vi "MCSControlPanel.vi"(4 "Register Map\nDefaults":refnum<vi>, 5 "StatusWord0x10Ref":refnum<vi>, 6 "Register Map\nRead Ref":refnum<vi>, 7 "NewRegMapReady":refnum<vi>, 8 "Last Command\nSent Ref":refnum<vi>, 9 "Stop Loop \nRef":refnum<vi>, 10 "error out":errorcluster, 11 "queue out":refnum<queue>) -> ()   [LabVIEW 2012]
panel:
  out "0x10 Status Word Readout":bool[][](array[boolean])
  in  "SYNC In \nVolt Threshold":u16
  out "word33":string
  in  "DIN In Volt \nThreshold":u16
  out "word32":string
  in  "DEMUX In Volt \nThreshold":u16
  out "word31":string
  in  "Power Mon Volt \nRef Threshold":u16
  out "word30":string
  out "wordB":string
  in  "Power Mon In 5 \nDEMUX Select":string(combo)
  in  "Power Mon In 4 \nDEMUX Select":string(combo)
  in  "Power Mon In 3 \nDEMUX Select":string(combo)
  in  "Power Mon In 2 \nDEMUX Select":string(combo)
  in  "Power Mon In 1 \nDEMUX Select":string(combo)
  in  "Power Mon In 0 \nDEMUX Select":string(combo)
  in  "Power Pulse\nReject Config":u16
  in  "Power Mon \nAcc Mode":string(combo)
  in  "Power Mon \nTest Mode":string(combo)
  in  "Power Mon Chan Enable   \n  11    10      9      8       7       6      5       4       3       2      1       0":bool[](array[boolean])
  out "word9":string
  in  "SoftDEMUX \nSelector Enable":bool
  in  "Sync Select 3B":string(combo)
  in  "Sync Select 2B":string(combo)
  in  "Sync Select 1B":string(combo)
  in  "Sync Select 0B":string(combo)
  in  "Sync Select 7":string(combo)
  in  "Sync Select 6":string(combo)
  in  "Sync Select 5":string(combo)
  in  "Sync Select 4":string(combo)
  in  "Sync Select 3A":string(combo)
  in  "Sync Select 2A":string(combo)
  in  "Sync Select 1A":string(combo)
  in  "Sync Select 0A":string(combo)
  in  "Sync Test\nMode Config":u32
  in  "Pulse Period\n(clock cycles -1)":u32
  in  "Channel DEMUX \nSelector":bool
  in  "Channel \nHold Order":bool
  in  "Channel \nTransfer Order":bool
  in  "Throttle Mode":string(combo)
  in  "Sync Test Mode Select":string(combo)
  in  "Data Input Test Mode":string(combo)
  out "Last Command Sent":string
  in  "Send Command, \nmanual entry":string
  in  "Send":bool
  in  "Reset Register Map\nto Defaults":bool
  in  "Sync Enable\n  2       1       0":bool[](array[boolean])
  in  "Channel Enable\n 11     10      9      8       7       6      5        4      3       2       1       0":bool[](array[boolean])
  in  "Reset Profile Accumulator  \n  11     10     9      8       7       6      5       4       3      2       1       0":bool[](array[boolean])
  in  "Counts Per Bin":u16
  in  "User Reset":bool
  in  "Number of Bins":u16
  in  "Profiles Per Histogram":u16
  in  "Time Reset":bool
  in  "Relative Time Step":u32
  in  "Demux Channel Enable\n  3       2       1      0":bool[](array[boolean])
  out "word0":string
  out "word1":string
  out "word2":string
  out "word3":string
  out "word4":string
  out "word5":string
  out "word6":string
  out "word7":string
  out "word8":string
  in  "DIN Polarity \n  7      6        5      4       3       2      1       0":bool[](array[boolean])
  in  "DIN Demux Polarity\n  3       2       1      0":bool[](array[boolean])
  in  "Sync Input Polarity\n  2       1       0":bool[](array[boolean])
  in  "PIN0 Pulse \nDurration Ave 2^N":u16
  out "wordA":string
  in  "PIN1 Pulse \nDurration Ave 2^N":u16
  in  "PIN2 Pulse \nDurration Ave 2^N":u16
  in  "PIN3 Pulse \nDurration Ave 2^N":u16
  in  "PIN4 Pulse \nDurration Ave 2^N":u16
  in  "PIN5 Pulse \nDurration Ave 2^N":u16
  # "word00"
  # "word30"
  # "valid range (0-65535)"
  # "word01"
  # "word02"
  # "word03"
  # "word04"
  # "word31"
  # "valid range (2-4095)"
  # "valid range (2-4095)"
  # "valid range (1-32,767)"
  # "valid range (0-65535)"
  # "word32"
  # "word05"
  # "valid range (0-65535)"
  # "7\n15\n23\n31"
  # "0\n8\n16\n24"
  # "word33"
  # "word06"
  # "valid range (0-65535)"
  # "valid range (0-255)"
  # "valid range (0-63)"
  # "word07"
  # "word08"
  # "word09"
  # "valid range (0-33,554,431)"
  # "valid range (0-256)"
  # "word0A"
  # "word0B"
  # "Expert Use Only"
  # "N=valid range (0-15)"
  # "N=valid range (0-15)"
  # "N=valid range (0-15)"
  # "N=valid range (0-15)"
  # "N=valid range (0-15)"
  # "N=valid range (0-15)"
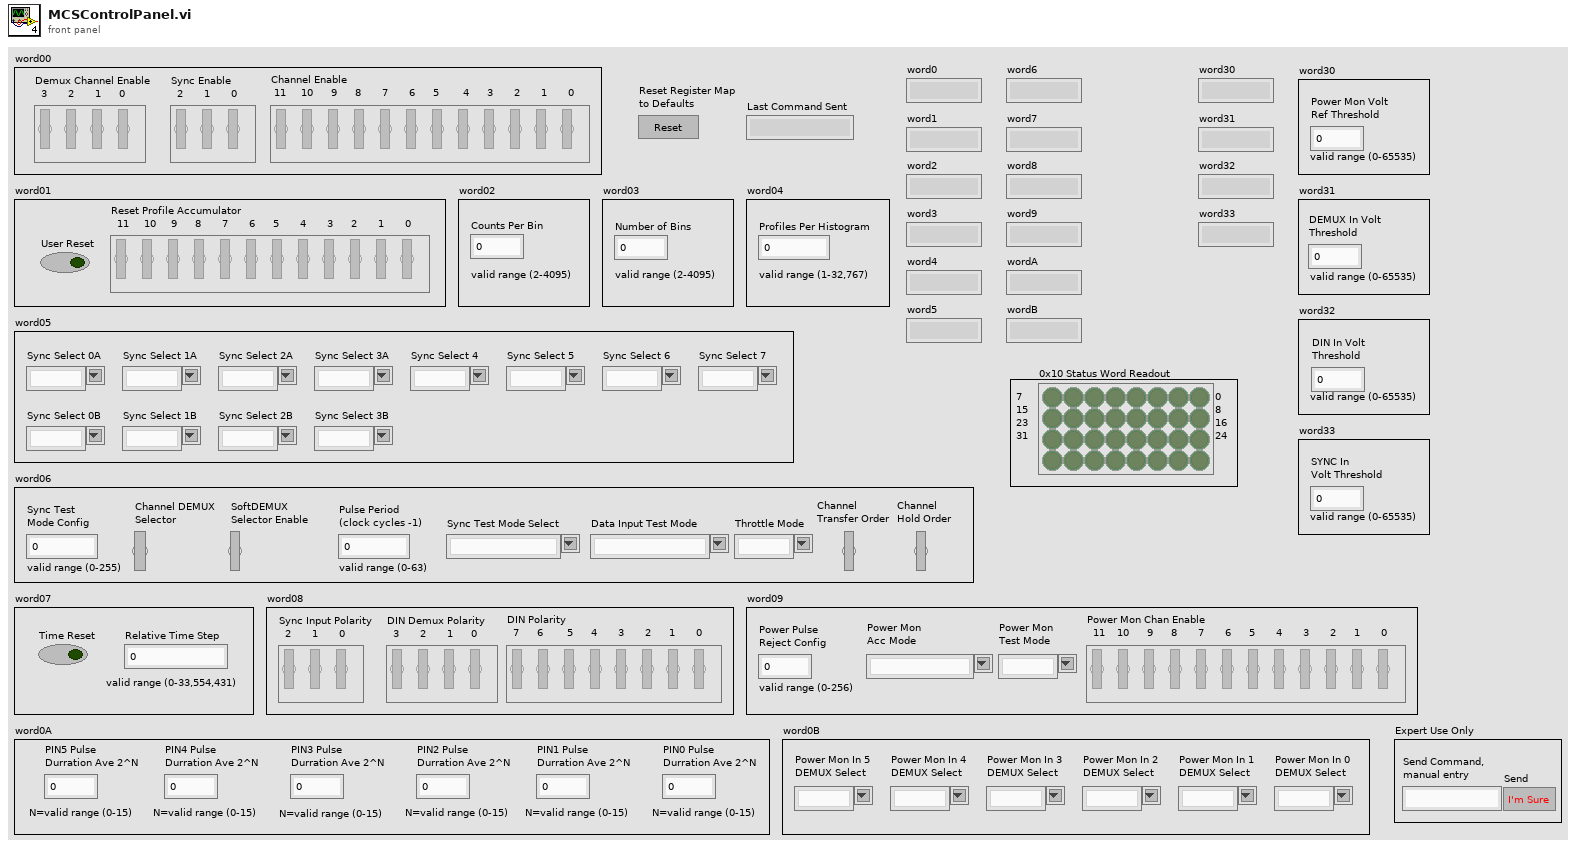
[diagram p1: front panel]
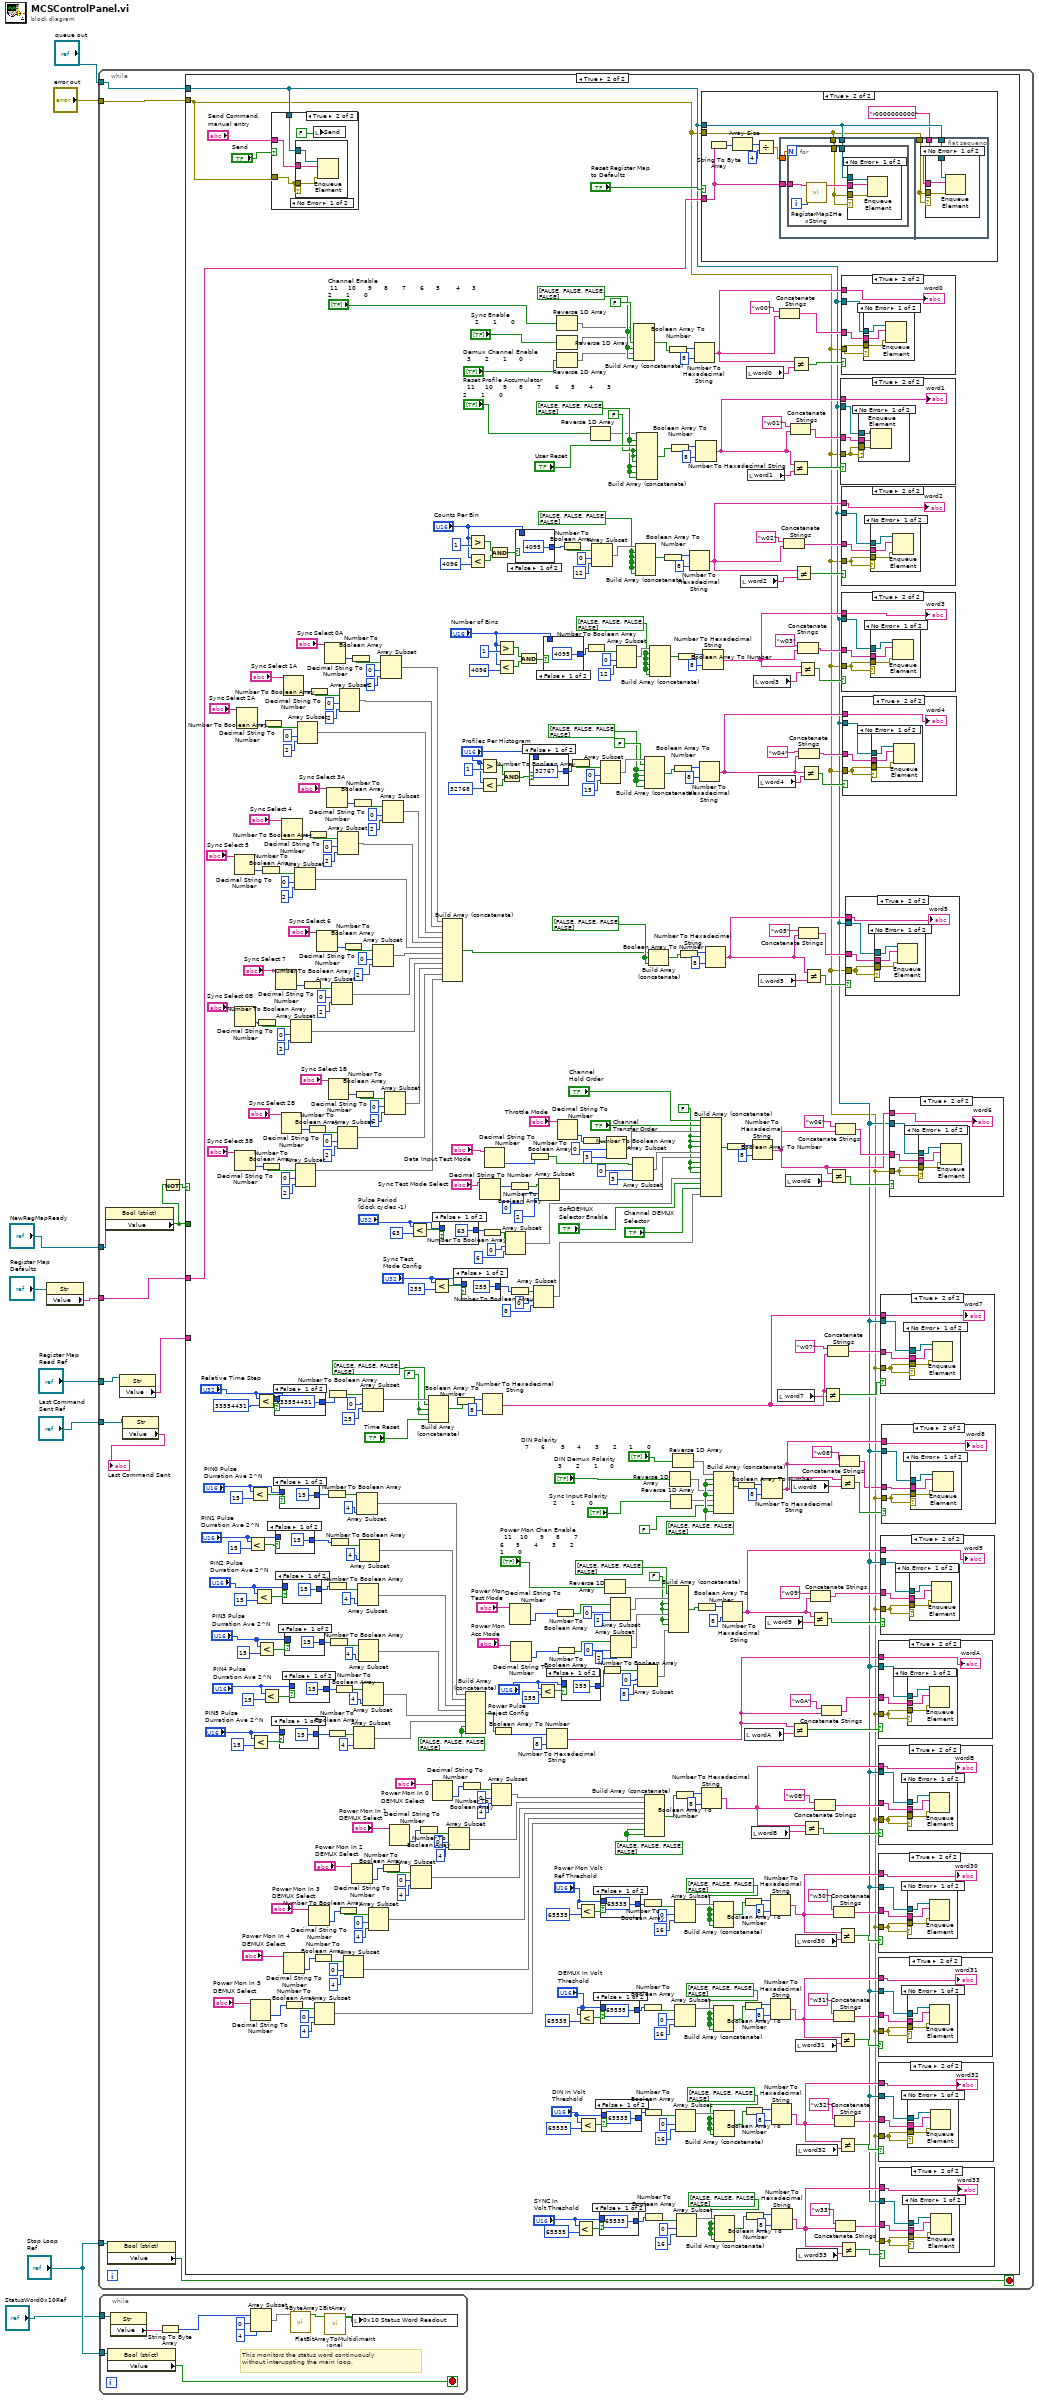
[diagram p0: block diagram]
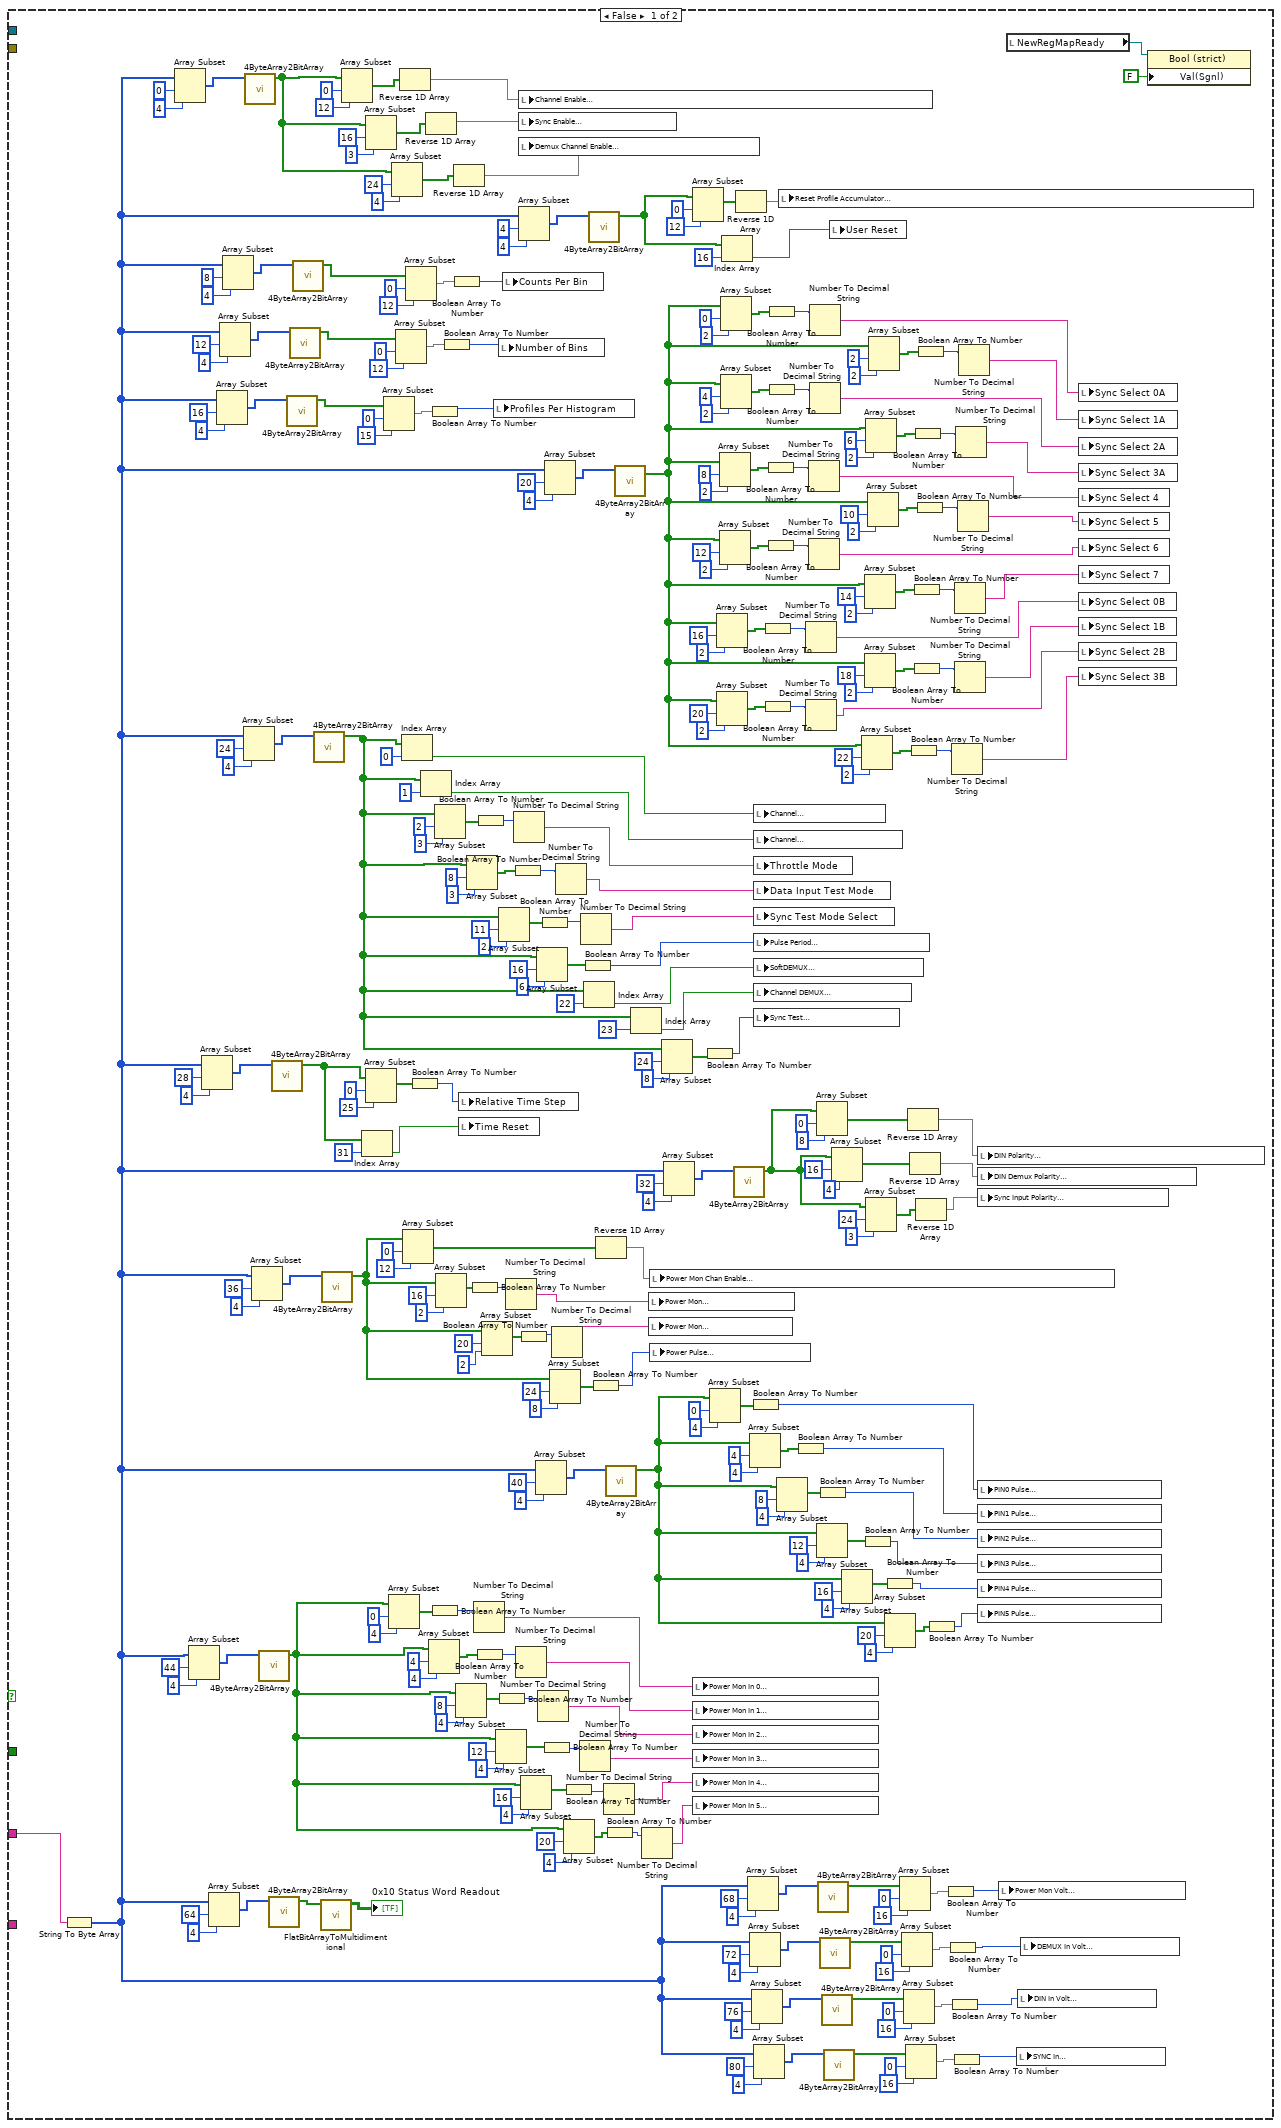
[diagram p2: hidden frame]
diagram:
  n1 = property class="Str"(reference="Register Map\nDefaults") -> ("Value"=w3:string)  [unwired: 1 in, 2 out]
  n2 = while {
    tunnel: "queue out" -> [w21]
    tunnel: "error out" -> [w20]
    tunnel: "Stop Loop \nRef" -> [w19]
    tunnel: "Last Command\nSent Ref" -> [w15]
    tunnel: "Register Map\nRead Ref" -> [w16]
    tunnel: w3 -> [w12]
    tunnel: "NewRegMapReady" -> [w13]
    stop <- w18 stop-if-true
    n3 = property class="Bool (strict)"(reference=w13) -> ("Value"=w10:bool)  [unwired: 1 in, 2 out]
    n4 = property class="Bool (strict)"(reference=w19) -> ("Value"=w18:bool)  [unwired: 1 in, 2 out]
    n5 = property class="Str"(reference=w16) -> ("Value"=w14:string)  [unwired: 1 in, 2 out]
    n6 = property class="Str"(reference=w15) -> ("Value"=→"Last Command Sent":string)  [unwired: 1 in, 2 out]
    n7 = Not(x=w10) -> (.not. x?=w11:bool)
    n8 = case shown="True" w11 {
      tunnel: w21 -> [_ w409]
      tunnel: w20 -> [_ w337]
      tunnel: w14 -> [_ _]
      tunnel: w12 -> [w44 w578]
      tunnel: w10 -> [_ _]
      frame False {
        n9 = String To Byte Array(string=w44) -> (unsigned byte array=w41:u8[])
        n10 = Array Subset(array=w41, index=0, length=4) -> (w290:u8[])
        n11 = Array Subset(array=w41, index=44, length=4) -> (w108:u8[])
        n12 = Array Subset(array=w41, index=28, length=4) -> (w296:u8[])
        n13 = Array Subset(array=w41, index=64, length=4) -> (w40:u8[])
        n14 = Array Subset(array=w41, index=16, length=4) -> (w305:u8[])
        n15 = Array Subset(array=w41, index=12, length=4) -> (w308:u8[])
        n16 = Array Subset(array=w41, index=8, length=4) -> (w311:u8[])
        n17 = Array Subset(array=w41, index=24, length=4) -> (w299:u8[])
        n18 = call "4ByteArray2BitArray.vi"("array"=w290) -> ("Array"=w136:bool[])  [unwired: 10 in]
        n19 = Array Subset(array=w41, index=36, length=4) -> (w130:u8[])
        n20 = call "4ByteArray2BitArray.vi"("array"=w108) -> ("Array"=w89:bool[])  [unwired: 10 in]
        n21 = call "4ByteArray2BitArray.vi"("array"=w40) -> ("Array"=w25:bool[])  [unwired: 10 in]
        n22 = call "4ByteArray2BitArray.vi"("array"=w296) -> ("Array"=w255:bool[])  [unwired: 10 in]
        n23 = call "4ByteArray2BitArray.vi"("array"=w305) -> ("Array"=w157:bool[])  [unwired: 10 in]
        n24 = call "4ByteArray2BitArray.vi"("array"=w308) -> ("Array"=w152:bool[])  [unwired: 10 in]
        n25 = call "4ByteArray2BitArray.vi"("array"=w311) -> ("Array"=w147:bool[])  [unwired: 10 in]
        n26 = call "4ByteArray2BitArray.vi"("array"=w299) -> ("Array"=w135:bool[])  [unwired: 10 in]
        n27 = call "FlatBitArrayToMultidimentional.vi"("Array in"=w25) -> ("Array out"=→"0x10 Status Word Readout":bool[][])  [unwired: 10 in]
        n28 = call "4ByteArray2BitArray.vi"("array"=w130) -> ("Array"=w117:bool[])  [unwired: 10 in]
        n29 = Array Subset(array=w136, index=0, length=12) -> (w38:bool[])
        n30 = Index Array(array=w255, index=31) -> (element=w253:bool)
        n31 = Array Subset(array=w136, index=16, length=3) -> (w36:bool[])
        n32 = Array Subset(array=w255, index=0, length=25) -> (w251:bool[])
        n33 = Array Subset(array=w157, index=0, length=15) -> (w158:bool[])
        n34 = Array Subset(array=w89, index=0, length=4) -> (w94:bool[])
        n35 = Array Subset(array=w136, index=24, length=4) -> (w34:bool[])
        n36 = Array Subset(array=w152, index=0, length=12) -> (w153:bool[])
        n37 = Reverse 1D Array(array=w38) -> (reversed array=w39:bool[])
        n38 = Index Array(array=w135, index=0) -> (element=w233:bool)
        n39 = Array Subset(array=w117, index=0, length=12) -> (w26:bool[])
        n40 = Array Subset(array=w147, index=0, length=12) -> (w148:bool[])
        n41 = Boolean Array To Number(Boolean array=w251) -> (number=w252:u32)
        n42 = Index Array(array=w135, index=1) -> (element=w232:bool)
        n43 = Reverse 1D Array(array=w36) -> (reversed array=w37:bool[])
        n44 = Array Subset(array=w89, index=4, length=4) -> (w95:bool[])
        n45 = Boolean Array To Number(Boolean array=w158) -> (number=w156:u32)
        n46 = Boolean Array To Number(Boolean array=w94) -> (number=w88:u32)
        n47 = Array Subset(array=w135, index=2, length=3) -> (w239:bool[])
        n48 = Array Subset(array=w117, index=16, length=2) -> (w126:bool[])
        n49 = Boolean Array To Number(Boolean array=w153) -> (number=w151:u32)
        n50 = Boolean Array To Number(Boolean array=w148) -> (number=w146:u32)
        n51 = Reverse 1D Array(array=w34) -> (reversed array=w35:bool[])
        n52 = Array Subset(array=w89, index=8, length=4) -> (w93:bool[])
        n53 = local write "Relative Time Step"(w252) -> ()
        n54 = local write "Time Reset"(w253) -> ()
        n55 = Array Subset(array=w135, index=8, length=3) -> (w240:bool[])
        n56 = Boolean Array To Number(Boolean array=w126) -> (number=w125:u32)
        n57 = Number To Decimal String(number=w88) -> (decimal integer string=w77:string)  [unwired: 1 in]
        n58 = Boolean Array To Number(Boolean array=w95) -> (number=w87:u32)
        n59 = Boolean Array To Number(Boolean array=w239) -> (number=w231:u32)
        n60 = Array Subset(array=w117, index=20, length=2) -> (w122:bool[])
        n61 = local write "Profiles Per Histogram"(w156) -> ()
        n62 = Array Subset(array=w89, index=12, length=4) -> (w92:bool[])
        n63 = Boolean Array To Number(Boolean array=w93) -> (number=w86:u32)
        n64 = local write "Number of Bins"(w151) -> ()
        n65 = Array Subset(array=w135, index=11, length=2) -> (w238:bool[])
        n66 = local write "Counts Per Bin"(w146) -> ()
        n67 = Number To Decimal String(number=w125) -> (decimal integer string=w124:string)  [unwired: 1 in]
        n68 = Boolean Array To Number(Boolean array=w240) -> (number=w229:u32)
        n69 = Number To Decimal String(number=w231) -> (decimal integer string=w230:string)  [unwired: 1 in]
        n70 = Number To Decimal String(number=w87) -> (decimal integer string=w78:string)  [unwired: 1 in]
        n71 = local write "Channel Enable\n 11     10      9      8       7       6      5        4      3       2       1       0"(w39) -> ()
        n72 = local write "Sync Enable\n  2       1       0"(w37) -> ()
        n73 = local write "Demux Channel Enable\n  3       2       1      0"(w35) -> ()
        n74 = Array Subset(array=w41, index=4, length=4) -> (w314:u8[])
        n75 = Boolean Array To Number(Boolean array=w122) -> (number=w121:u32)
        n76 = Array Subset(array=w89, index=16, length=4) -> (w91:bool[])
        n77 = Array Subset(array=w41, index=40, length=4) -> (w317:u8[])
        n78 = Array Subset(array=w135, index=16, length=6) -> (w237:bool[])
        n79 = Number To Decimal String(number=w86) -> (decimal integer string=w79:string)  [unwired: 1 in]
        n80 = Boolean Array To Number(Boolean array=w238) -> (number=w227:u32)
        n81 = Boolean Array To Number(Boolean array=w92) -> (number=w84:u32)
        n82 = Array Subset(array=w41, index=20, length=4) -> (w302:u8[])
        n83 = Array Subset(array=w117, index=24, length=8) -> (w118:bool[])
        n84 = Number To Decimal String(number=w121) -> (decimal integer string=w120:string)  [unwired: 1 in]
        n85 = Number To Decimal String(number=w229) -> (decimal integer string=w228:string)  [unwired: 1 in]
        n86 = Boolean Array To Number(Boolean array=w91) -> (number=w85:u32)
        n87 = Array Subset(array=w89, index=20, length=4) -> (w90:bool[])
        n88 = Number To Decimal String(number=w84) -> (decimal integer string=w80:string)  [unwired: 1 in]
        n89 = Number To Decimal String(number=w227) -> (decimal integer string=w226:string)  [unwired: 1 in]
        n90 = Boolean Array To Number(Boolean array=w237) -> (number=w223:u32)
        n91 = Index Array(array=w135, index=22) -> (element=w133:bool)
        n92 = call "4ByteArray2BitArray.vi"("array"=w314) -> ("Array"=w142:bool[])  [unwired: 10 in]
        n93 = Boolean Array To Number(Boolean array=w118) -> (number=w116:u32)
        n94 = Reverse 1D Array(array=w26) -> (reversed array=w27:bool[])
        n95 = Number To Decimal String(number=w85) -> (decimal integer string=w81:string)  [unwired: 1 in]
        n96 = Boolean Array To Number(Boolean array=w90) -> (number=w83:u32)
        n97 = call "4ByteArray2BitArray.vi"("array"=w317) -> ("Array"=w277:bool[])  [unwired: 10 in]
        n98 = call "4ByteArray2BitArray.vi"("array"=w302) -> ("Array"=w173:bool[])  [unwired: 10 in]
        n99 = Index Array(array=w135, index=23) -> (element=w224:bool)
        n100 = Number To Decimal String(number=w83) -> (decimal integer string=w82:string)  [unwired: 1 in]
        n101 = local write "Power Mon \nTest Mode"(w124) -> ()
        n102 = local write "Power Mon \nAcc Mode"(w120) -> ()
        n103 = local write "Power Mon Chan Enable   \n  11    10      9      8       7       6      5       4       3       2      1       0"(w27) -> ()
        n104 = local write "Power Pulse\nReject Config"(w116) -> ()
        n105 = Array Subset(array=w135, index=24, length=8) -> (w236:bool[])
        n106 = Array Subset(array=w41, index=32, length=4) -> (w293:u8[])
        n107 = Array Subset(array=w142, index=0, length=12) -> (w32:bool[])
        n108 = local write "Power Mon In 0 \nDEMUX Select"(w77) -> ()
        n109 = local write "Power Mon In 1 \nDEMUX Select"(w78) -> ()
        n110 = local write "Power Mon In 2 \nDEMUX Select"(w79) -> ()
        n111 = local write "Power Mon In 3 \nDEMUX Select"(w80) -> ()
        n112 = local write "Power Mon In 4 \nDEMUX Select"(w81) -> ()
        n113 = local write "Power Mon In 5 \nDEMUX Select"(w82) -> ()
        n114 = Boolean Array To Number(Boolean array=w236) -> (number=w222:u32)
        n115 = Array Subset(array=w277, index=0, length=4) -> (w274:bool[])
        n116 = Array Subset(array=w173, index=16, length=2) -> (w187:bool[])
        n117 = Array Subset(array=w173, index=20, length=2) -> (w179:bool[])
        n118 = Array Subset(array=w173, index=8, length=2) -> (w203:bool[])
        n119 = Array Subset(array=w173, index=12, length=2) -> (w195:bool[])
        n120 = Array Subset(array=w173, index=0, length=2) -> (w219:bool[])
        n121 = Array Subset(array=w173, index=4, length=2) -> (w211:bool[])
        n122 = Index Array(array=w142, index=16) -> (element=w141:bool)
        n123 = call "4ByteArray2BitArray.vi"("array"=w293) -> ("Array"=w258:bool[])  [unwired: 10 in]
        n124 = Reverse 1D Array(array=w32) -> (reversed array=w33:bool[])
        n125 = Array Subset(array=w41, index=68, length=4) -> (w74:u8[])
        n126 = Array Subset(array=w277, index=4, length=4) -> (w276:bool[])
        n127 = Array Subset(array=w41, index=72, length=4) -> (w67:u8[])
        n128 = Boolean Array To Number(Boolean array=w274) -> (number=w273:u32)
        n129 = Array Subset(array=w41, index=76, length=4) -> (w60:u8[])
        n130 = local write "Channel \nHold Order"(w233) -> ()
        n131 = local write "Channel \nTransfer Order"(w232) -> ()
        n132 = local write "Throttle Mode"(w230) -> ()
        n133 = local write "Data Input Test Mode"(w228) -> ()
        n134 = local write "Sync Test Mode Select"(w226) -> ()
        n135 = local write "Pulse Period\n(clock cycles -1)"(w223) -> ()
        n136 = local write "SoftDEMUX \nSelector Enable"(w133) -> ()
        n137 = local write "Channel DEMUX \nSelector"(w224) -> ()
        n138 = local write "Sync Test\nMode Config"(w222) -> ()
        n139 = Array Subset(array=w41, index=80, length=4) -> (w53:u8[])
        n140 = Boolean Array To Number(Boolean array=w187) -> (number=w186:u32)
        n141 = Boolean Array To Number(Boolean array=w179) -> (number=w178:u32)
        n142 = Boolean Array To Number(Boolean array=w203) -> (number=w202:u32)
        n143 = Boolean Array To Number(Boolean array=w195) -> (number=w194:u32)
        n144 = Boolean Array To Number(Boolean array=w219) -> (number=w218:u32)
        n145 = Boolean Array To Number(Boolean array=w211) -> (number=w210:u32)
        n146 = Array Subset(array=w277, index=8, length=4) -> (w271:bool[])
        n147 = local write "Reset Profile Accumulator  \n  11     10     9      8       7       6      5       4       3      2       1       0"(w33) -> ()
        n148 = Boolean Array To Number(Boolean array=w276) -> (number=w275:u32)
        n149 = Number To Decimal String(number=w186) -> (decimal integer string=w164:string)  [unwired: 1 in]
        n150 = Number To Decimal String(number=w178) -> (decimal integer string=w162:string)  [unwired: 1 in]
        n151 = Number To Decimal String(number=w202) -> (decimal integer string=w168:string)  [unwired: 1 in]
        n152 = Number To Decimal String(number=w194) -> (decimal integer string=w166:string)  [unwired: 1 in]
        n153 = Number To Decimal String(number=w218) -> (decimal integer string=w172:string)  [unwired: 1 in]
        n154 = Number To Decimal String(number=w210) -> (decimal integer string=w170:string)  [unwired: 1 in]
        n155 = Array Subset(array=w258, index=0, length=8) -> (w28:bool[])
        n156 = Array Subset(array=w277, index=12, length=4) -> (w270:bool[])
        n157 = Boolean Array To Number(Boolean array=w271) -> (number=w272:u32)
        n158 = call "4ByteArray2BitArray.vi"("array"=w74) -> ("Array"=w70:bool[])  [unwired: 10 in]
        n159 = call "4ByteArray2BitArray.vi"("array"=w67) -> ("Array"=w63:bool[])  [unwired: 10 in]
        n160 = call "4ByteArray2BitArray.vi"("array"=w60) -> ("Array"=w56:bool[])  [unwired: 10 in]
        n161 = call "4ByteArray2BitArray.vi"("array"=w53) -> ("Array"=w49:bool[])  [unwired: 10 in]
        n162 = local write "User Reset"(w141) -> ()
        n163 = Array Subset(array=w258, index=16, length=4) -> (w29:bool[])
        n164 = Array Subset(array=w277, index=16, length=4) -> (w269:bool[])
        n165 = Array Subset(array=w173, index=22, length=2) -> (w175:bool[])
        n166 = Boolean Array To Number(Boolean array=w270) -> (number=w265:u32)
        n167 = Array Subset(array=w173, index=14, length=2) -> (w191:bool[])
        n168 = Array Subset(array=w173, index=18, length=2) -> (w183:bool[])
        n169 = Array Subset(array=w173, index=6, length=2) -> (w207:bool[])
        n170 = Array Subset(array=w258, index=24, length=3) -> (w30:bool[])
        n171 = Array Subset(array=w173, index=10, length=2) -> (w199:bool[])
        n172 = Array Subset(array=w173, index=2, length=2) -> (w215:bool[])
        n173 = Boolean Array To Number(Boolean array=w269) -> (number=w266:u32)
        n174 = Array Subset(array=w277, index=20, length=4) -> (w268:bool[])
        n175 = Array Subset(array=w70, index=0, length=16) -> (w71:bool[])
        n176 = Array Subset(array=w63, index=0, length=16) -> (w64:bool[])
        n177 = Array Subset(array=w56, index=0, length=16) -> (w57:bool[])
        n178 = Array Subset(array=w49, index=0, length=16) -> (w50:bool[])
        n179 = Reverse 1D Array(array=w28) -> (reversed array=w31:bool[])
        n180 = Boolean Array To Number(Boolean array=w175) -> (number=w174:u32)
        n181 = Reverse 1D Array(array=w29) -> (reversed array=w23:bool[])
        n182 = Boolean Array To Number(Boolean array=w191) -> (number=w190:u32)
        n183 = Boolean Array To Number(Boolean array=w183) -> (number=w182:u32)
        n184 = Boolean Array To Number(Boolean array=w207) -> (number=w206:u32)
        n185 = Boolean Array To Number(Boolean array=w199) -> (number=w198:u32)
        n186 = Boolean Array To Number(Boolean array=w215) -> (number=w214:u32)
        n187 = Reverse 1D Array(array=w30) -> (reversed array=w22:bool[])
        n188 = Boolean Array To Number(Boolean array=w268) -> (number=w267:u32)
        n189 = Boolean Array To Number(Boolean array=w71) -> (number=w48:u32)
        n190 = Boolean Array To Number(Boolean array=w64) -> (number=w47:u32)
        n191 = Boolean Array To Number(Boolean array=w57) -> (number=w46:u32)
        n192 = Number To Decimal String(number=w174) -> (decimal integer string=w161:string)  [unwired: 1 in]
        n193 = Boolean Array To Number(Boolean array=w50) -> (number=w45:u32)
        n194 = Number To Decimal String(number=w190) -> (decimal integer string=w165:string)  [unwired: 1 in]
        n195 = Number To Decimal String(number=w182) -> (decimal integer string=w163:string)  [unwired: 1 in]
        n196 = Number To Decimal String(number=w206) -> (decimal integer string=w169:string)  [unwired: 1 in]
        n197 = Number To Decimal String(number=w198) -> (decimal integer string=w167:string)  [unwired: 1 in]
        n198 = Number To Decimal String(number=w214) -> (decimal integer string=w171:string)  [unwired: 1 in]
        n199 = local write "DIN Polarity \n  7      6        5      4       3       2      1       0"(w31) -> ()
        n200 = local write "DIN Demux Polarity\n  3       2       1      0"(w23) -> ()
        n201 = local write "Sync Input Polarity\n  2       1       0"(w22) -> ()
        n202 = local write "PIN0 Pulse \nDurration Ave 2^N"(w273) -> ()
        n203 = local write "PIN1 Pulse \nDurration Ave 2^N"(w275) -> ()
        n204 = local write "PIN2 Pulse \nDurration Ave 2^N"(w272) -> ()
        n205 = local write "PIN3 Pulse \nDurration Ave 2^N"(w265) -> ()
        n206 = local write "PIN4 Pulse \nDurration Ave 2^N"(w266) -> ()
        n207 = local write "PIN5 Pulse \nDurration Ave 2^N"(w267) -> ()
        n208 = local write "Power Mon Volt \nRef Threshold"(w48) -> ()
        n209 = local read "NewRegMapReady"() -> (w112:refnum<vi>)
        n210 = local write "SYNC In \nVolt Threshold"(w45) -> ()
        n211 = local write "DIN In Volt \nThreshold"(w46) -> ()
        n212 = local write "DEMUX In Volt \nThreshold"(w47) -> ()
        n213 = local write "Sync Select 0A"(w172) -> ()
        n214 = local write "Sync Select 1A"(w171) -> ()
        n215 = local write "Sync Select 2A"(w170) -> ()
        n216 = local write "Sync Select 3A"(w169) -> ()
        n217 = local write "Sync Select 4"(w168) -> ()
        n218 = local write "Sync Select 5"(w167) -> ()
        n219 = local write "Sync Select 6"(w166) -> ()
        n220 = local write "Sync Select 7"(w165) -> ()
        n221 = local write "Sync Select 0B"(w164) -> ()
        n222 = local write "Sync Select 1B"(w163) -> ()
        n223 = local write "Sync Select 2B"(w162) -> ()
        n224 = local write "Sync Select 3B"(w161) -> ()
        n225 = property class="Bool (strict)"(reference=w112, "Val(Sgnl)"=FALSE ("Value (Signaling)")) -> ()  [unwired: 1 in, 2 out]
      }
      frame True {
        w410 = bool[] [FALSE, FALSE, FALSE, FALSE] ("appended array")
        w423 = bool[] [FALSE, FALSE, FALSE, FALSE] ("appended array")
        w436 = bool[] [FALSE, FALSE, FALSE, FALSE] ("appended array")
        w449 = bool[] [FALSE, FALSE, FALSE, FALSE] ("appended array")
        w508 = bool[] [FALSE, FALSE, FALSE, FALSE] ("appended array")
        w407 = FALSE ("Read Register")
        w726 = bool[] [FALSE, FALSE, FALSE, FALSE] ("appended array")
        w744 = bool[] [FALSE, FALSE, FALSE, FALSE] ("appended array")
        w746 = FALSE ("Read Register")
        w687 = FALSE ("Read Register")
        w751 = bool[] [FALSE, FALSE, FALSE, FALSE] ("appended array")
        w610 = bool[] [FALSE, FALSE, FALSE, FALSE] ("appended array")
        w749 = bool[] [FALSE, FALSE, FALSE, FALSE] ("appended array")
        w750 = bool[] [FALSE, FALSE, FALSE, FALSE] ("appended array")
        w762 = FALSE ("Read Register")
        w761 = bool[] [FALSE, FALSE, FALSE, FALSE] ("appended array")
        w764 = bool[] [FALSE, FALSE, FALSE, FALSE] ("appended array")
        n226 = Decimal String To Number(string="Sync Select 5") -> (number=w654:i32)  [unwired: 2 in, 1 out]
        n227 = Decimal String To Number(string="Sync Select 0B") -> (number=w639:i32)  [unwired: 2 in, 1 out]
        n228 = Decimal String To Number(string="Sync Select 3B") -> (number=w624:i32)  [unwired: 2 in, 1 out]
        n229 = Decimal String To Number(string="Sync Select 2A") -> (number=w669:i32)  [unwired: 2 in, 1 out]
        n230 = Less?(x="PIN1 Pulse \nDurration Ave 2^N", y=u16 15) -> (x < y?=w371:bool)
        n231 = Less?(x="PIN0 Pulse \nDurration Ave 2^N", y=u16 15) -> (x < y?=w377:bool)
        n232 = Decimal String To Number(string="Power Mon In 5 \nDEMUX Select") -> (number=w511:i32)  [unwired: 2 in, 1 out]
        n233 = Less?(x="PIN5 Pulse \nDurration Ave 2^N", y=u16 15) -> (x < y?=w382:bool)
        n234 = Less?(x="PIN2 Pulse \nDurration Ave 2^N", y=u16 15) -> (x < y?=w375:bool)
        n235 = Less?(x="Relative Time Step", y=u64 33554431) -> (x < y?=w339:bool)
        n236 = Number To Boolean Array(number=w639) -> (Boolean array=w641:bool[])
        n237 = Less?(x="PIN3 Pulse \nDurration Ave 2^N", y=u16 15) -> (x < y?=w373:bool)
        n238 = Number To Boolean Array(number=w654) -> (Boolean array=w656:bool[])
        n239 = Number To Boolean Array(number=w624) -> (Boolean array=w626:bool[])
        n240 = Less?(x="PIN4 Pulse \nDurration Ave 2^N", y=u16 15) -> (x < y?=w379:bool)
        n241 = Number To Boolean Array(number=w669) -> (Boolean array=w671:bool[])
        n242 = case shown="True" "Send" {
          tunnel: "Send Command, \nmanual entry" -> [_ w953]
          tunnel: w409 -> [_ w952]
          tunnel: w337 -> [_ w950]
          frame False {
          }
          frame True {
            n243 = case shown="No Error" w950 {
              tunnel: w953 -> [w956 _]
              tunnel: w950 -> [w955 _]
              tunnel: w952 -> [w954 _]
              frame No Error {
                n244 = Enqueue Element(queue=w954, element=w956, error in (no error)=w955) -> ()  [unwired: 1 in, 3 out]
              }
              frame Error {
              }
            }
            n245 = local write "Send"(FALSE ("Send")) -> ()
          }
        }
        n246 = case shown="False" w339 {
          tunnel: [u64 33554431 ("Counts Per Bin") w783] -> w328
          tunnel: "Relative Time Step" -> [_ w783]
          frame False {
          }
          frame True {
          }
        }
        n247 = case shown="False" w371 {
          tunnel: [u16 15 ("Counts Per Bin") w795] -> w364
          tunnel: "PIN1 Pulse \nDurration Ave 2^N" -> [_ w795]
          frame False {
          }
          frame True {
          }
        }
        n248 = Decimal String To Number(string="Sync Select 7") -> (number=w644:i32)  [unwired: 2 in, 1 out]
        n249 = case shown="False" w382 {
          tunnel: [u16 15 ("Counts Per Bin") w805] -> w383
          tunnel: "PIN5 Pulse \nDurration Ave 2^N" -> [_ w805]
          frame False {
          }
          frame True {
          }
        }
        n250 = case shown="False" w377 {
          tunnel: [u16 15 ("Counts Per Bin") w801] -> w361
          tunnel: "PIN0 Pulse \nDurration Ave 2^N" -> [_ w801]
          frame False {
          }
          frame True {
          }
        }
        n251 = Decimal String To Number(string="Sync Select 2B") -> (number=w629:i32)  [unwired: 2 in, 1 out]
        n252 = Decimal String To Number(string="Sync Select 4") -> (number=w659:i32)  [unwired: 2 in, 1 out]
        n253 = case shown="False" w375 {
          tunnel: [u16 15 ("Counts Per Bin") w799] -> w366
          tunnel: "PIN2 Pulse \nDurration Ave 2^N" -> [_ w799]
          frame False {
          }
          frame True {
          }
        }
        n254 = Decimal String To Number(string="Sync Select 1A") -> (number=w674:i32)  [unwired: 2 in, 1 out]
        n255 = Decimal String To Number(string="Power Mon In 4 \nDEMUX Select") -> (number=w521:i32)  [unwired: 2 in, 1 out]
        n256 = Number To Boolean Array(number=w511) -> (Boolean array=w512:bool[])
        n257 = case shown="False" w373 {
          tunnel: [u16 15 ("Counts Per Bin") w797] -> w368
          tunnel: "PIN3 Pulse \nDurration Ave 2^N" -> [_ w797]
          frame False {
          }
          frame True {
          }
        }
        n258 = case shown="False" w379 {
          tunnel: [u16 15 ("Counts Per Bin") w803] -> w369
          tunnel: "PIN4 Pulse \nDurration Ave 2^N" -> [_ w803]
          frame False {
          }
          frame True {
          }
        }
        n259 = Array Subset(array=w641, index=0, length=2) -> (w614:bool[])
        n260 = Array Subset(array=w656, index=0, length=2) -> (w618:bool[])
        n261 = Array Subset(array=w626, index=0, length=2) -> (w617:bool[])
        n262 = Array Subset(array=w671, index=0, length=2) -> (w621:bool[])
        n263 = Number To Boolean Array(number=w644) -> (Boolean array=w646:bool[])
        n264 = Number To Boolean Array(number=w629) -> (Boolean array=w631:bool[])
        n265 = Number To Boolean Array(number=w659) -> (Boolean array=w661:bool[])
        n266 = Decimal String To Number(string="Power Mon In 3 \nDEMUX Select") -> (number=w526:i32)  [unwired: 2 in, 1 out]
        n267 = Number To Boolean Array(number=w674) -> (Boolean array=w676:bool[])
        n268 = Number To Boolean Array(number=w521) -> (Boolean array=w522:bool[])
        n269 = Array Subset(array=w512, index=0, length=4) -> (w509:bool[])
        n270 = Decimal String To Number(string="Sync Select 6") -> (number=w649:i32)  [unwired: 2 in, 1 out]
        n271 = Decimal String To Number(string="Sync Select 0A") -> (number=w679:i32)  [unwired: 2 in, 1 out]
        n272 = Decimal String To Number(string="Sync Select 3A") -> (number=w664:i32)  [unwired: 2 in, 1 out]
        n273 = Number To Boolean Array(number=w361) -> (Boolean array=w742:bool[])
        n274 = Number To Boolean Array(number=w383) -> (Boolean array=w736:bool[])
        n275 = Number To Boolean Array(number=w328) -> (Boolean array=w766:bool[])
        n276 = Number To Boolean Array(number=w366) -> (Boolean array=w732:bool[])
        n277 = Decimal String To Number(string="Sync Select 1B") -> (number=w634:i32)  [unwired: 2 in, 1 out]
        n278 = Number To Boolean Array(number=w368) -> (Boolean array=w734:bool[])
        n279 = Number To Boolean Array(number=w364) -> (Boolean array=w740:bool[])
        n280 = Array Subset(array=w646, index=0, length=2) -> (w613:bool[])
        n281 = Number To Boolean Array(number=w369) -> (Boolean array=w738:bool[])
        n282 = Array Subset(array=w631, index=0, length=2) -> (w616:bool[])
        n283 = Array Subset(array=w661, index=0, length=2) -> (w619:bool[])
        n284 = Number To Boolean Array(number=w526) -> (Boolean array=w527:bool[])
        n285 = Array Subset(array=w676, index=0, length=2) -> (w622:bool[])
        n286 = Number To Boolean Array(number=w649) -> (Boolean array=w651:bool[])
        n287 = Array Subset(array=w522, index=0, length=4) -> (w515:bool[])
        n288 = Number To Boolean Array(number=w679) -> (Boolean array=w681:bool[])
        n289 = Decimal String To Number(string="Power Mon In 2 \nDEMUX Select") -> (number=w531:i32)  [unwired: 2 in, 1 out]
        n290 = Number To Boolean Array(number=w664) -> (Boolean array=w666:bool[])
        n291 = Array Subset(array=w736, length=4) -> (w727:bool[])  [unwired: 1 in]
        n292 = Number To Boolean Array(number=w634) -> (Boolean array=w636:bool[])
        n293 = Array Subset(array=w742, length=4) -> (w385:bool[])  [unwired: 1 in]
        n294 = Array Subset(array=w732, length=4) -> (w730:bool[])  [unwired: 1 in]
        n295 = Array Subset(array=w734, length=4) -> (w729:bool[])  [unwired: 1 in]
        n296 = Array Subset(array=w740, length=4) -> (w731:bool[])  [unwired: 1 in]
        n297 = Array Subset(array=w766, index=0, length=25) -> (w748:bool[])
        n298 = Array Subset(array=w738, length=4) -> (w728:bool[])  [unwired: 1 in]
        n299 = Array Subset(array=w527, index=0, length=4) -> (w516:bool[])
        n300 = Array Subset(array=w651, index=0, length=2) -> (w612:bool[])
        n301 = Array Subset(array=w681, index=0, length=2) -> (w623:bool[])
        n302 = Number To Boolean Array(number=w531) -> (Boolean array=w532:bool[])
        n303 = Array Subset(array=w666, index=0, length=2) -> (w620:bool[])
        n304 = Array Subset(array=w636, index=0, length=2) -> (w615:bool[])
        n305 = Decimal String To Number(string="Power Mon In 1 \nDEMUX Select") -> (number=w536:i32)  [unwired: 2 in, 1 out]
        n306 = Less?(x="Pulse Period\n(clock cycles -1)", y=u16 63) -> (x < y?=w335:bool)
        n307 = Array Subset(array=w532, index=0, length=4) -> (w517:bool[])
        n308 = Number To Boolean Array(number=w536) -> (Boolean array=w537:bool[])
        n309 = Build Array (concatenate)(w748, bool[] [FALSE, FALSE, FALSE, FALSE] ("appended array"), w746, w746, "Time Reset") -> (w581:bool[])
        n310 = Less?(x="Sync Test\nMode Config", y=u16 255) -> (x < y?=w332:bool)
        n311 = Decimal String To Number(string="Power Mon In 0 \nDEMUX Select") -> (number=w541:i32)  [unwired: 2 in, 1 out]
        n312 = case shown="False" w335 {
          tunnel: [u16 63 ("Counts Per Bin") w781] -> w329
          tunnel: "Pulse Period\n(clock cycles -1)" -> [_ w781]
          frame False {
          }
          frame True {
          }
        }
        n313 = Build Array (concatenate)(w623, w622, w621, w620, w619, w618, w612, w613, w614, w615, w616, w617) -> (w708:bool[])
        n314 = Array Subset(array=w537, index=0, length=4) -> (w518:bool[])
        n315 = Boolean Array To Number(Boolean array=w581) -> (number=w593:u32)
        n316 = case shown="False" w332 {
          tunnel: [u16 255 ("Counts Per Bin") w779] -> w331
          tunnel: "Sync Test\nMode Config" -> [_ w779]
          frame False {
          }
          frame True {
          }
        }
        n317 = Number To Boolean Array(number=w541) -> (Boolean array=w542:bool[])
        n318 = Build Array (concatenate)(w385, w731, w730, w729, w728, w727, w726, w726) -> (w579:bool[])
        n319 = Greater?(x="Counts Per Bin", y=u16 1) -> (0:w403:bool)
        n320 = Less?(x="Counts Per Bin", y=u16 4096) -> (x < y?=w402:bool)
        n321 = Greater?(x="Profiles Per Histogram", y=u16 1) -> (0:w390:bool)
        n322 = Less?(x="Profiles Per Histogram", y=u16 32768) -> (x < y?=w389:bool)
        n323 = Decimal String To Number(string="Sync Test Mode Select") -> (number=w702:i32)  [unwired: 2 in, 1 out]
        n324 = Number To Boolean Array(number=w329) -> (Boolean array=w695:bool[])
        n325 = Number To Hexadecimal String(1:i16 8 ("width (-)"), 2:w593) -> (0:w499:string)
        n326 = Decimal String To Number(string="Data Input Test Mode") -> (number=w703:i32)  [unwired: 2 in, 1 out]
        n327 = And(x=w403, y=w402) -> (x .and. y?=w404:bool)
        n328 = Array Subset(array=w542, index=0, length=4) -> (w519:bool[])
        n329 = Boolean Array To Number(Boolean array=w579) -> (number=w589:u32)
        n330 = Greater?(x="Number of Bins", y=u16 1) -> (0:w396:bool)
        n331 = Less?(x="Number of Bins", y=u16 4096) -> (x < y?=w395:bool)
        n332 = And(x=w390, y=w389) -> (x .and. y?=w391:bool)
        n333 = Array Subset(array=w695, index=0, length=6) -> (w576:bool[])
        n334 = Number To Boolean Array(number=w702) -> (Boolean array=w696:bool[])
        n335 = Number To Boolean Array(number=w331) -> (Boolean array=w686:bool[])
        n336 = Decimal String To Number(string="Power Mon \nTest Mode") -> (number=w565:i32)  [unwired: 2 in, 1 out]
        n337 = Decimal String To Number(string="Power Mon \nAcc Mode") -> (number=w560:i32)  [unwired: 2 in, 1 out]
        n338 = case shown="False" w404 {
          tunnel: [u16 4095 ("Counts Per Bin") w811] -> w400
          tunnel: "Counts Per Bin" -> [_ w811]
          frame False {
          }
          frame True {
          }
        }
        n339 = And(x=w396, y=w395) -> (x .and. y?=w397:bool)
        n340 = case shown="False" w391 {
          tunnel: [u16 32767 ("Counts Per Bin") w807] -> w387
          tunnel: "Profiles Per Histogram" -> [_ w807]
          frame False {
          }
          frame True {
          }
        }
        n341 = Number To Boolean Array(number=w703) -> (Boolean array=w697:bool[])
        n342 = Array Subset(array=w686, index=0, length=8) -> (w577:bool[])
        n343 = Less?(x="Power Pulse\nReject Config", y=u16 255) -> (x < y?=w345:bool)
        n344 = Array Subset(array=w696, index=0, length=2) -> (w688:bool[])
        n345 = case shown="False" w397 {
          tunnel: [u16 4095 ("Counts Per Bin") w809] -> w327
          tunnel: "Number of Bins" -> [_ w809]
          frame False {
          }
          frame True {
          }
        }
        n346 = Number To Hexadecimal String(1:i16 8 ("width (-)"), 2:w589) -> (0:w341:string)
        n347 = Number To Boolean Array(number=w565) -> (Boolean array=w564:bool[])
        n348 = Number To Boolean Array(number=w560) -> (Boolean array=w559:bool[])
        n349 = Reverse 1D Array(array="Channel Enable\n 11     10      9      8       7       6      5        4      3       2       1       0") -> (reversed array=w465:bool[])
        n350 = Reverse 1D Array(array="Sync Enable\n  2       1       0") -> (reversed array=w466:bool[])
        n351 = Reverse 1D Array(array="Demux Channel Enable\n  3       2       1      0") -> (reversed array=w467:bool[])
        n352 = Decimal String To Number(string="Throttle Mode") -> (number=w706:i32)  [unwired: 2 in, 1 out]
        n353 = case shown="False" w345 {
          tunnel: [u16 255 ("Counts Per Bin") w785] -> w344
          tunnel: "Power Pulse\nReject Config" -> [_ w785]
          frame False {
          }
          frame True {
          }
        }
        n354 = Number To Boolean Array(number=w400) -> (Boolean array=w772:bool[])
        n355 = Number To Boolean Array(number=w387) -> (Boolean array=w753:bool[])
        n356 = Less?(x="SYNC In \nVolt Threshold", y=u16 65535) -> (x < y?=w359:bool)
        n357 = Less?(x="DEMUX In Volt \nThreshold", y=u16 65535) -> (x < y?=w351:bool)
        n358 = Less?(x="Power Mon Volt \nRef Threshold", y=u16 65535) -> (x < y?=w355:bool)
        n359 = Less?(x="DIN In Volt \nThreshold", y=u16 65535) -> (x < y?=w353:bool)
        n360 = Number To Boolean Array(number=w706) -> (Boolean array=w769:bool[])
        n361 = Number To Boolean Array(number=w327) -> (Boolean array=w757:bool[])
        n362 = Reverse 1D Array(array="Reset Profile Accumulator  \n  11     10     9      8       7       6      5       4       3      2       1       0") -> (reversed array=w468:bool[])
        n363 = Array Subset(array=w772, index=0, length=12) -> (w760:bool[])
        n364 = case shown="False" w359 {
          tunnel: [u16 65535 ("Counts Per Bin") w793] -> w358
          tunnel: "SYNC In \nVolt Threshold" -> [_ w793]
          frame False {
          }
          frame True {
          }
        }
        n365 = Array Subset(array=w753, index=0, length=15) -> (w752:bool[])
        n366 = case shown="False" w351 {
          tunnel: [u16 65535 ("Counts Per Bin") w787] -> w325
          tunnel: "DEMUX In Volt \nThreshold" -> [_ w787]
          frame False {
          }
          frame True {
          }
        }
        n367 = case shown="False" w355 {
          tunnel: [u16 65535 ("Counts Per Bin") w791] -> w326
          tunnel: "Power Mon Volt \nRef Threshold" -> [_ w791]
          frame False {
          }
          frame True {
          }
        }
        n368 = case shown="False" w353 {
          tunnel: [u16 65535 ("Counts Per Bin") w789] -> w350
          tunnel: "DIN In Volt \nThreshold" -> [_ w789]
          frame False {
          }
          frame True {
          }
        }
        n369 = Number To Boolean Array(number=w344) -> (Boolean array=w554:bool[])
        n370 = Reverse 1D Array(array="Power Mon Chan Enable   \n  11    10      9      8       7       6      5       4       3       2      1       0") -> (reversed array=w474:bool[])
        n371 = Array Subset(array=w769, index=0, length=3) -> (w692:bool[])
        n372 = Array Subset(array=w564, index=0, length=2) -> (w561:bool[])
        n373 = Array Subset(array=w559, index=0, length=2) -> (w408:bool[])
        n374 = Array Subset(array=w757, index=0, length=12) -> (w756:bool[])
        n375 = Array Subset(array=w697, index=0, length=3) -> (w689:bool[])
        n376 = Build Array (concatenate)(w465, w764, w466, FALSE ("Read Register"), w764, w467, w764) -> (w587:bool[])
        n377 = Build Array (concatenate)(w760, w750, w750, w750, w750, w750) -> (w585:bool[])
        n378 = Build Array (concatenate)(w468, w761, "User Reset", w762, w762, w762, w761, w761, w761) -> (w586:bool[])
        n379 = Array Subset(array=w554, index=0, length=8) -> (w406:bool[])
        n380 = Number To Boolean Array(number=w326) -> (Boolean array=w451:bool[])
        n381 = Number To Boolean Array(number=w325) -> (Boolean array=w438:bool[])
        n382 = Number To Boolean Array(number=w350) -> (Boolean array=w425:bool[])
        n383 = Number To Boolean Array(number=w358) -> (Boolean array=w412:bool[])
        n384 = Build Array (concatenate)(w752, FALSE ("Read Register"), w610, w610, w610, w610) -> (w584:bool[])
        n385 = Build Array (concatenate)(w519, w518, w517, w516, w515, w509, w508, w508) -> (w549:bool[])
        n386 = Build Array (concatenate)(w708, w751, w751) -> (w583:bool[])
        n387 = Build Array (concatenate)(w756, w749, w749, w749, w749, w749) -> (w606:bool[])
        n388 = Boolean Array To Number(Boolean array=w585) -> (number=w601:u32)
        n389 = Boolean Array To Number(Boolean array=w587) -> (number=w605:u32)
        n390 = Build Array (concatenate)(w474, bool[] [FALSE, FALSE, FALSE, FALSE] ("appended array"), w561, w407, w407, w408, w407, w407, w406) -> (w568:bool[])
        n391 = Boolean Array To Number(Boolean array=w586) -> (number=w603:u32)
        n392 = Reverse 1D Array(array="DIN Demux Polarity\n  3       2       1      0") -> (reversed array=w324:bool[])
        n393 = Reverse 1D Array(array="Sync Input Polarity\n  2       1       0") -> (reversed array=w323:bool[])
        n394 = Boolean Array To Number(Boolean array=w584) -> (number=w599:u32)
        n395 = Reverse 1D Array(array="DIN Polarity \n  7      6        5      4       3       2      1       0") -> (reversed array=w473:bool[])
        n396 = Boolean Array To Number(Boolean array=w549) -> (number=w551:u32)
        n397 = Array Subset(array=w451, index=0, length=16) -> (w450:bool[])
        n398 = Array Subset(array=w438, index=0, length=16) -> (w437:bool[])
        n399 = Array Subset(array=w425, index=0, length=16) -> (w424:bool[])
        n400 = Boolean Array To Number(Boolean array=w606) -> (number=w608:u32)
        n401 = Array Subset(array=w412, index=0, length=16) -> (w411:bool[])
        n402 = Boolean Array To Number(Boolean array=w583) -> (number=w597:u32)
        n403 = Number To Hexadecimal String(1:i16 8 ("width (-)"), 2:w601) -> (0:w484:string)
        n404 = Number To Hexadecimal String(1:i16 8 ("width (-)"), 2:w605) -> (0:w477:string)
        n405 = Number To Hexadecimal String(1:i16 8 ("width (-)"), 2:w603) -> (0:w481:string)
        n406 = Boolean Array To Number(Boolean array=w568) -> (number=w570:u32)
        n407 = Number To Hexadecimal String(1:i16 8 ("width (-)"), 2:w599) -> (0:w488:string)
        n408 = Build Array (concatenate)("Channel \nHold Order", "Channel \nTransfer Order", w692, w687, w687, w687, w689, w688, w687, w687, w687, w576, "SoftDEMUX \nSelector Enable", "Channel DEMUX \nSelector", w577) -> (w582:bool[])
        n409 = case shown="True" "Reset Register Map\nto Defaults" {
          tunnel: w409 -> [_ w926]
          tunnel: w337 -> [_ w925]
          tunnel: w578 -> [_ w931]
          frame False {
          }
          frame True {
            n410 = String To Byte Array(string=w931) -> (unsigned byte array=w930:u8[])
            n411 = Array Size(array=w930) -> (size(s)=w928:i32)
            n412 = Divide(x=w928, y=4) -> (x/y=w929:dbl)
            n413 = flat-sequence {
              tunnel: w926 -> [w935]
              tunnel: w925 -> [w934]
              tunnel: w931 -> [w933]
              tunnel: w929 -> [w932]
              tunnel: w926 -> [w946]
              tunnel: w925 -> [w945]
              tunnel: "r0000000000" ("data in") -> [w944]
              frame #0 {
                n414 = for {
                  N: w932 -> [_]
                  tunnel: w935 -> [w939]
                  tunnel: w934 -> [w938]
                  tunnel: w933 -> [w937]
                  i -> [w936]
                  n415 = call "RegisterMap2HexString.vi"("Word Num"=w936, "string"=w937) -> ("concatenated string"=w940:string)  [unwired: 9 in]
                  n416 = case shown="No Error" w938 {
                    tunnel: w939 -> [w943 _]
                    tunnel: w938 -> [w942 _]
                    tunnel: w940 -> [w941 _]
                    frame No Error {
                      n417 = Enqueue Element(queue=w943, element=w941, error in (no error)=w942) -> ()  [unwired: 1 in, 3 out]
                    }
                    frame Error {
                    }
                  }
                }
              }
              frame #1 {
                n418 = case shown="No Error" w945 {
                  tunnel: w945 -> [w949 _]
                  tunnel: w944 -> [w948 _]
                  tunnel: w946 -> [w947 _]
                  frame No Error {
                    n419 = Enqueue Element(queue=w947, element=w948, error in (no error)=w949) -> ()  [unwired: 1 in, 3 out]
                  }
                  frame Error {
                  }
                }
              }
            }
          }
        }
        n420 = Number To Hexadecimal String(1:i16 8 ("width (-)"), 2:w551) -> (0:w546:string)
        n421 = Number To Hexadecimal String(1:i16 8 ("width (-)"), 2:w608) -> (0:w486:string)
        n422 = Number To Hexadecimal String(1:i16 8 ("width (-)"), 2:w597) -> (0:w493:string)
        n423 = Build Array (concatenate)(w473, w744, w744, w324, w744, w323, FALSE ("Read Register"), w744) -> (w580:bool[])
        n424 = Build Array (concatenate)(w450, w449, w449, w449, w449) -> (w458:bool[])
        n425 = Build Array (concatenate)(w437, w436, w436, w436, w436) -> (w445:bool[])
        n426 = Build Array (concatenate)(w424, w423, w423, w423, w423) -> (w432:bool[])
        n427 = Build Array (concatenate)(w411, w410, w410, w410, w410) -> (w419:bool[])
        n428 = Number To Hexadecimal String(1:i16 8 ("width (-)"), 2:w570) -> (0:w503:string)
        n429 = Boolean Array To Number(Boolean array=w582) -> (number=w595:u32)
        n430 = Boolean Array To Number(Boolean array=w580) -> (number=w591:u32)
        n431 = local read "word2"() -> (w482:string)
        n432 = Boolean Array To Number(Boolean array=w458) -> (number=w460:u32)
        n433 = Boolean Array To Number(Boolean array=w445) -> (number=w447:u32)
        n434 = Boolean Array To Number(Boolean array=w432) -> (number=w434:u32)
        n435 = local read "wordA"() -> (w507:string)
        n436 = Boolean Array To Number(Boolean array=w419) -> (number=w421:u32)
        n437 = local read "word0"() -> (w476:string)
        n438 = local read "word1"() -> (w480:string)
        n439 = local read "wordB"() -> (w548:string)
        n440 = Number To Hexadecimal String(1:i16 8 ("width (-)"), 2:w595) -> (0:w496:string)
        n441 = local read "word3"() -> (w485:string)
        n442 = local read "word4"() -> (w489:string)
        n443 = local read "word5"() -> (w492:string)
        n444 = Number To Hexadecimal String(1:i16 8 ("width (-)"), 2:w591) -> (0:w501:string)
        n445 = local read "word9"() -> (w505:string)
        n446 = Number To Hexadecimal String(1:i16 8 ("width (-)"), 2:w460) -> (0:w455:string)
        n447 = Number To Hexadecimal String(1:i16 8 ("width (-)"), 2:w447) -> (0:w442:string)
        n448 = Number To Hexadecimal String(1:i16 8 ("width (-)"), 2:w434) -> (0:w429:string)
        n449 = Number To Hexadecimal String(1:i16 8 ("width (-)"), 2:w421) -> (0:w416:string)
        n450 = local read "word7"() -> (w498:string)
        n451 = Concatenate Strings("w00" ("string"), w477) -> (w724:string)
        n452 = Concatenate Strings("w02" ("string"), w484) -> (w713:string)
        n453 = local read "word6"() -> (w494:string)
        n454 = Concatenate Strings("w01" ("string"), w481) -> (w714:string)
        n455 = Not Equal?(x=w481, y=w480) -> (x != y?=w479:bool)
        n456 = Not Equal?(x=w341, y=w507) -> (x != y?=w506:bool)
        n457 = Not Equal?(x=w477, y=w476) -> (x != y?=w478:bool)
        n458 = local read "word8"() -> (w502:string)
        n459 = Not Equal?(x=w484, y=w482) -> (x != y?=w483:bool)
        n460 = local read "word30"() -> (w457:string)
        n461 = local read "word31"() -> (w444:string)
        n462 = local read "word32"() -> (w431:string)
        n463 = local read "word33"() -> (w418:string)
        n464 = Concatenate Strings("w03" ("string"), w486) -> (w609:string)
        n465 = Not Equal?(x=w486, y=w485) -> (x != y?=w487:bool)
        n466 = Concatenate Strings("w05" ("string"), w493) -> (w711:string)
        n467 = Concatenate Strings("w04" ("string"), w488) -> (w712:string)
        n468 = Not Equal?(x=w488, y=w489) -> (x != y?=w490:bool)
        n469 = Not Equal?(x=w546, y=w548) -> (x != y?=w545:bool)
        n470 = Not Equal?(x=w493, y=w492) -> (x != y?=w491:bool)
        n471 = Concatenate Strings("w09" ("string"), w503) -> (w571:string)
        n472 = Not Equal?(x=w503, y=w505) -> (x != y?=w504:bool)
        n473 = Concatenate Strings("w0B" ("string"), w546) -> (w547:string)
        n474 = Concatenate Strings("w0A" ("string"), w341) -> (w573:string)
        n475 = Not Equal?(x=w499, y=w498) -> (x != y?=w497:bool)
        n476 = Concatenate Strings("w07" ("string"), w499) -> (w709:string)
        n477 = Not Equal?(x=w496, y=w494) -> (x != y?=w495:bool)
        n478 = Concatenate Strings("w30" ("string"), w455) -> (w456:string)
        n479 = Concatenate Strings("w31" ("string"), w442) -> (w443:string)
        n480 = Concatenate Strings("w32" ("string"), w429) -> (w430:string)
        n481 = Concatenate Strings("w06" ("string"), w496) -> (w710:string)
        n482 = Concatenate Strings("w33" ("string"), w416) -> (w417:string)
        n483 = Not Equal?(x=w455, y=w457) -> (x != y?=w454:bool)
        n484 = Not Equal?(x=w442, y=w444) -> (x != y?=w441:bool)
        n485 = Not Equal?(x=w501, y=w502) -> (x != y?=w500:bool)
        n486 = Not Equal?(x=w429, y=w431) -> (x != y?=w428:bool)
        n487 = Not Equal?(x=w416, y=w418) -> (x != y?=w415:bool)
        n488 = Concatenate Strings("w08" ("string"), w501) -> (w342:string)
        n489 = case shown="True" w479 {
          tunnel: w714 -> [_ w913]
          tunnel: w409 -> [_ w911]
          tunnel: w337 -> [_ w912]
          tunnel: w481 -> [_ w910]
          frame False {
          }
          frame True {
            n490 = case shown="No Error" w912 {
              tunnel: w913 -> [w916 _]
              tunnel: w912 -> [w915 _]
              tunnel: w911 -> [w914 _]
              frame No Error {
                n491 = Enqueue Element(queue=w914, element=w916, error in (no error)=w915) -> ()  [unwired: 1 in, 3 out]
              }
              frame Error {
              }
            }
            "word1" <- w910
          }
        }
        n492 = case shown="True" w478 {
          tunnel: w724 -> [_ w920]
          tunnel: w409 -> [_ w919]
          tunnel: w337 -> [_ w918]
          tunnel: w477 -> [_ w917]
          frame False {
          }
          frame True {
            n493 = case shown="No Error" w918 {
              tunnel: w920 -> [w923 _]
              tunnel: w918 -> [w922 _]
              tunnel: w919 -> [w921 _]
              frame No Error {
                n494 = Enqueue Element(queue=w921, element=w923, error in (no error)=w922) -> ()  [unwired: 1 in, 3 out]
              }
              frame Error {
              }
            }
            "word0" <- w917
          }
        }
        n495 = case shown="True" w483 {
          tunnel: w713 -> [_ w906]
          tunnel: w409 -> [_ w905]
          tunnel: w337 -> [_ w904]
          tunnel: w484 -> [_ w903]
          frame False {
          }
          frame True {
            n496 = case shown="No Error" w904 {
              tunnel: w906 -> [w909 _]
              tunnel: w904 -> [w908 _]
              tunnel: w905 -> [w907 _]
              frame No Error {
                n497 = Enqueue Element(queue=w907, element=w909, error in (no error)=w908) -> ()  [unwired: 1 in, 3 out]
              }
              frame Error {
              }
            }
            "word2" <- w903
          }
        }
        n498 = case shown="True" w487 {
          tunnel: w609 -> [_ w899]
          tunnel: w409 -> [_ w898]
          tunnel: w337 -> [_ w897]
          tunnel: w486 -> [_ w896]
          frame False {
          }
          frame True {
            n499 = case shown="No Error" w897 {
              tunnel: w899 -> [w902 _]
              tunnel: w897 -> [w901 _]
              tunnel: w898 -> [w900 _]
              frame No Error {
                n500 = Enqueue Element(queue=w900, element=w902, error in (no error)=w901) -> ()  [unwired: 1 in, 3 out]
              }
              frame Error {
              }
            }
            "word3" <- w896
          }
        }
        n501 = case shown="True" w490 {
          tunnel: w712 -> [_ w892]
          tunnel: w409 -> [_ w891]
          tunnel: w337 -> [_ w890]
          tunnel: w488 -> [_ w889]
          frame False {
          }
          frame True {
            n502 = case shown="No Error" w890 {
              tunnel: w892 -> [w895 _]
              tunnel: w890 -> [w894 _]
              tunnel: w891 -> [w893 _]
              frame No Error {
                n503 = Enqueue Element(queue=w893, element=w895, error in (no error)=w894) -> ()  [unwired: 1 in, 3 out]
              }
              frame Error {
              }
            }
            "word4" <- w889
          }
        }
        n504 = case shown="True" w491 {
          tunnel: w711 -> [_ w885]
          tunnel: w409 -> [_ w884]
          tunnel: w337 -> [_ w883]
          tunnel: w493 -> [_ w882]
          frame False {
          }
          frame True {
            n505 = case shown="No Error" w883 {
              tunnel: w885 -> [w888 _]
              tunnel: w883 -> [w887 _]
              tunnel: w884 -> [w886 _]
              frame No Error {
                n506 = Enqueue Element(queue=w886, element=w888, error in (no error)=w887) -> ()  [unwired: 1 in, 3 out]
              }
              frame Error {
              }
            }
            "word5" <- w882
          }
        }
        n507 = case shown="True" w506 {
          tunnel: w573 -> [_ w850]
          tunnel: w409 -> [_ w849]
          tunnel: w337 -> [_ w848]
          tunnel: w341 -> [_ w847]
          frame False {
          }
          frame True {
            n508 = case shown="No Error" w848 {
              tunnel: w850 -> [w853 _]
              tunnel: w848 -> [w852 _]
              tunnel: w849 -> [w851 _]
              frame No Error {
                n509 = Enqueue Element(queue=w851, element=w853, error in (no error)=w852) -> ()  [unwired: 1 in, 3 out]
              }
              frame Error {
              }
            }
            "wordA" <- w847
          }
        }
        n510 = case shown="True" w545 {
          tunnel: w547 -> [_ w843]
          tunnel: w409 -> [_ w842]
          tunnel: w337 -> [_ w841]
          tunnel: w546 -> [_ w840]
          frame False {
          }
          frame True {
            n511 = case shown="No Error" w841 {
              tunnel: w843 -> [w846 _]
              tunnel: w841 -> [w845 _]
              tunnel: w842 -> [w844 _]
              frame No Error {
                n512 = Enqueue Element(queue=w844, element=w846, error in (no error)=w845) -> ()  [unwired: 1 in, 3 out]
              }
              frame Error {
              }
            }
            "wordB" <- w840
          }
        }
        n513 = case shown="True" w454 {
          tunnel: w456 -> [_ w836]
          tunnel: w409 -> [_ w835]
          tunnel: w337 -> [_ w834]
          tunnel: w455 -> [_ w833]
          frame False {
          }
          frame True {
            n514 = case shown="No Error" w834 {
              tunnel: w836 -> [w839 _]
              tunnel: w834 -> [w838 _]
              tunnel: w835 -> [w837 _]
              frame No Error {
                n515 = Enqueue Element(queue=w837, element=w839, error in (no error)=w838) -> ()  [unwired: 1 in, 3 out]
              }
              frame Error {
              }
            }
            "word30" <- w833
          }
        }
        n516 = case shown="True" w441 {
          tunnel: w443 -> [_ w829]
          tunnel: w409 -> [_ w828]
          tunnel: w337 -> [_ w827]
          tunnel: w442 -> [_ w826]
          frame False {
          }
          frame True {
            n517 = case shown="No Error" w827 {
              tunnel: w829 -> [w832 _]
              tunnel: w827 -> [w831 _]
              tunnel: w828 -> [w830 _]
              frame No Error {
                n518 = Enqueue Element(queue=w830, element=w832, error in (no error)=w831) -> ()  [unwired: 1 in, 3 out]
              }
              frame Error {
              }
            }
            "word31" <- w826
          }
        }
        n519 = case shown="True" w428 {
          tunnel: w430 -> [_ w822]
          tunnel: w409 -> [_ w821]
          tunnel: w337 -> [_ w820]
          tunnel: w429 -> [_ w819]
          frame False {
          }
          frame True {
            n520 = case shown="No Error" w820 {
              tunnel: w822 -> [w825 _]
              tunnel: w820 -> [w824 _]
              tunnel: w821 -> [w823 _]
              frame No Error {
                n521 = Enqueue Element(queue=w823, element=w825, error in (no error)=w824) -> ()  [unwired: 1 in, 3 out]
              }
              frame Error {
              }
            }
            "word32" <- w819
          }
        }
        n522 = case shown="True" w415 {
          tunnel: w417 -> [_ w815]
          tunnel: w409 -> [_ w814]
          tunnel: w337 -> [_ w813]
          tunnel: w416 -> [_ w812]
          frame False {
          }
          frame True {
            n523 = case shown="No Error" w813 {
              tunnel: w815 -> [w818 _]
              tunnel: w813 -> [w817 _]
              tunnel: w814 -> [w816 _]
              frame No Error {
                n524 = Enqueue Element(queue=w816, element=w818, error in (no error)=w817) -> ()  [unwired: 1 in, 3 out]
              }
              frame Error {
              }
            }
            "word33" <- w812
          }
        }
        n525 = case shown="True" w504 {
          tunnel: w571 -> [_ w857]
          tunnel: w409 -> [_ w856]
          tunnel: w337 -> [_ w855]
          tunnel: w503 -> [_ w854]
          frame False {
          }
          frame True {
            n526 = case shown="No Error" w855 {
              tunnel: w857 -> [w860 _]
              tunnel: w855 -> [w859 _]
              tunnel: w856 -> [w858 _]
              frame No Error {
                n527 = Enqueue Element(queue=w858, element=w860, error in (no error)=w859) -> ()  [unwired: 1 in, 3 out]
              }
              frame Error {
              }
            }
            "word9" <- w854
          }
        }
        n528 = case shown="True" w497 {
          tunnel: w709 -> [_ w871]
          tunnel: w409 -> [_ w870]
          tunnel: w337 -> [_ w869]
          tunnel: w499 -> [_ w868]
          frame False {
          }
          frame True {
            n529 = case shown="No Error" w869 {
              tunnel: w871 -> [w874 _]
              tunnel: w869 -> [w873 _]
              tunnel: w870 -> [w872 _]
              frame No Error {
                n530 = Enqueue Element(queue=w872, element=w874, error in (no error)=w873) -> ()  [unwired: 1 in, 3 out]
              }
              frame Error {
              }
            }
            "word7" <- w868
          }
        }
        n531 = case shown="True" w500 {
          tunnel: w342 -> [_ w864]
          tunnel: w409 -> [_ w863]
          tunnel: w337 -> [_ w862]
          tunnel: w501 -> [_ w861]
          frame False {
          }
          frame True {
            n532 = case shown="No Error" w862 {
              tunnel: w864 -> [w867 _]
              tunnel: w862 -> [w866 _]
              tunnel: w863 -> [w865 _]
              frame No Error {
                n533 = Enqueue Element(queue=w865, element=w867, error in (no error)=w866) -> ()  [unwired: 1 in, 3 out]
              }
              frame Error {
              }
            }
            "word8" <- w861
          }
        }
        n534 = case shown="True" w495 {
          tunnel: w710 -> [_ w878]
          tunnel: w409 -> [_ w877]
          tunnel: w337 -> [_ w876]
          tunnel: w496 -> [_ w875]
          frame False {
          }
          frame True {
            n535 = case shown="No Error" w876 {
              tunnel: w878 -> [w881 _]
              tunnel: w876 -> [w880 _]
              tunnel: w877 -> [w879 _]
              frame No Error {
                n536 = Enqueue Element(queue=w879, element=w881, error in (no error)=w880) -> ()  [unwired: 1 in, 3 out]
              }
              frame Error {
              }
            }
            "word6" <- w875
          }
        }
      }
    }
  }
  n537 = while {
    tunnel: "Stop Loop \nRef" -> [w961]
    tunnel: "StatusWord0x10Ref" -> [w958]
    stop <- w960 stop-if-true
    # "This monitors the status word continuously\nwithout interuppting the main loop."
    n538 = property class="Bool (strict)"(reference=w961) -> ("Value"=w960:bool)  [unwired: 1 in, 2 out]
    n539 = property class="Str"(reference=w958) -> ("Value"=w959:string)  [unwired: 1 in, 2 out]
    n540 = String To Byte Array(string=w959) -> (unsigned byte array=w964:u8[])
    n541 = Array Subset(array=w964, index=0, length=4) -> (w963:u8[])
    n542 = call "4ByteArray2BitArray.vi"("array"=w963) -> ("Array"=w962:bool[])  [unwired: 10 in]
    n543 = call "FlatBitArrayToMultidimentional.vi"("Array in"=w962) -> ("Array out"=w957:bool[][])  [unwired: 10 in]
    n544 = local write "0x10 Status Word Readout"(w957) -> ()
  }
